vi "VI Snippet VI Tree.vi"   [LabVIEW 2019]
doc: "VI Tree for VI Snippet Import and Export API.\n\nCreated by: Ryan Pacini"
uses:
  VI Snippet.lvlib
panel:
  # "SEE DIAGRAM\nFOR VI Tree"
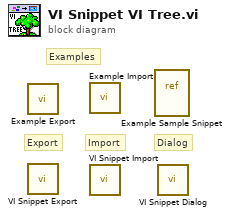
[diagram p0: block diagram]
diagram:
  # "Dialog"
  # "Examples"
  # "Import"
  # "Export"
  n1 = call "Example Export.vi"() -> ()  [unwired: 12 in]
  n2 = call "VI Snippet Export.vi"() -> ()  [unwired: 11 in, 1 out]
  n3 = call "Example Import.vi"() -> ()  [unwired: 12 in]
  n4 = call "VI Snippet Import.vi"() -> ()  [unwired: 8 in, 4 out]
  n5 = vi-ref "Example Sample Snippet.vi"() -> ()  [unwired: 1 out]
  n6 = call "VI Snippet Dialog.vi"() -> ()  [unwired: 8 in, 4 out]
